vi "Initialize.vi"(8 "error in (no error)":errorcluster, 10 "ConnectParameter":T1, 11 "DataBase in":refnum<class "DataBase.lvclass">) -> (0 "error out":errorcluster, 3 "DataBase out":refnum<class "DataBase.lvclass">)   [LabVIEW 2019, in "DataBase.lvlib" / "DataBase.lvclass"]
uses:
  DataBase.lvclass
  C:/Program Files (x86)/National Instruments/LabVIEW 2019/vi.lib/NI/Event Source Actor/Event Source/Event Source/Event Source.lvclass
  MySQL initial error.lvclass
  C:/Program Files (x86)/National Instruments/LabVIEW 2019/vi.lib/NI/Event Source Actor/Event Source/Event/Event.lvclass
  <vilib>/NI/Event Source Actor/Event Source/Event/Event.lvclass/Event.ctl
  DataBase.lvclass/DataBase.ctl
  <vilib>/addons/database/Connection.llb/DB Tools Open Connec (String).vi
  <vilib>/addons/database/NI_Database_API.lvlib
  <vilib>/NI/Event Source Actor/Event Source/Event/Event.lvclass
  <vilib>/NI/Event Source Actor/Event Source/Event Source/Event Source.lvclass
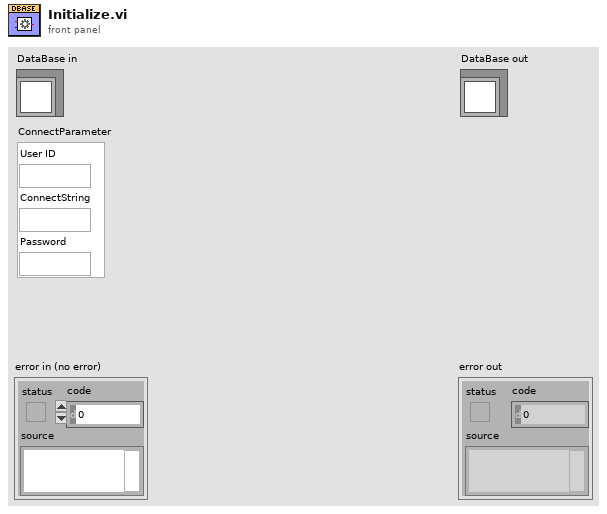
[diagram p1: front panel]
types:
  T1 = cluster{"User ID":string, "ConnectString":string, "Password":string}
  T2 = typedef "NI_Database_API.lvlib/Conn ObjectReference.ctl" = refnum<k1>
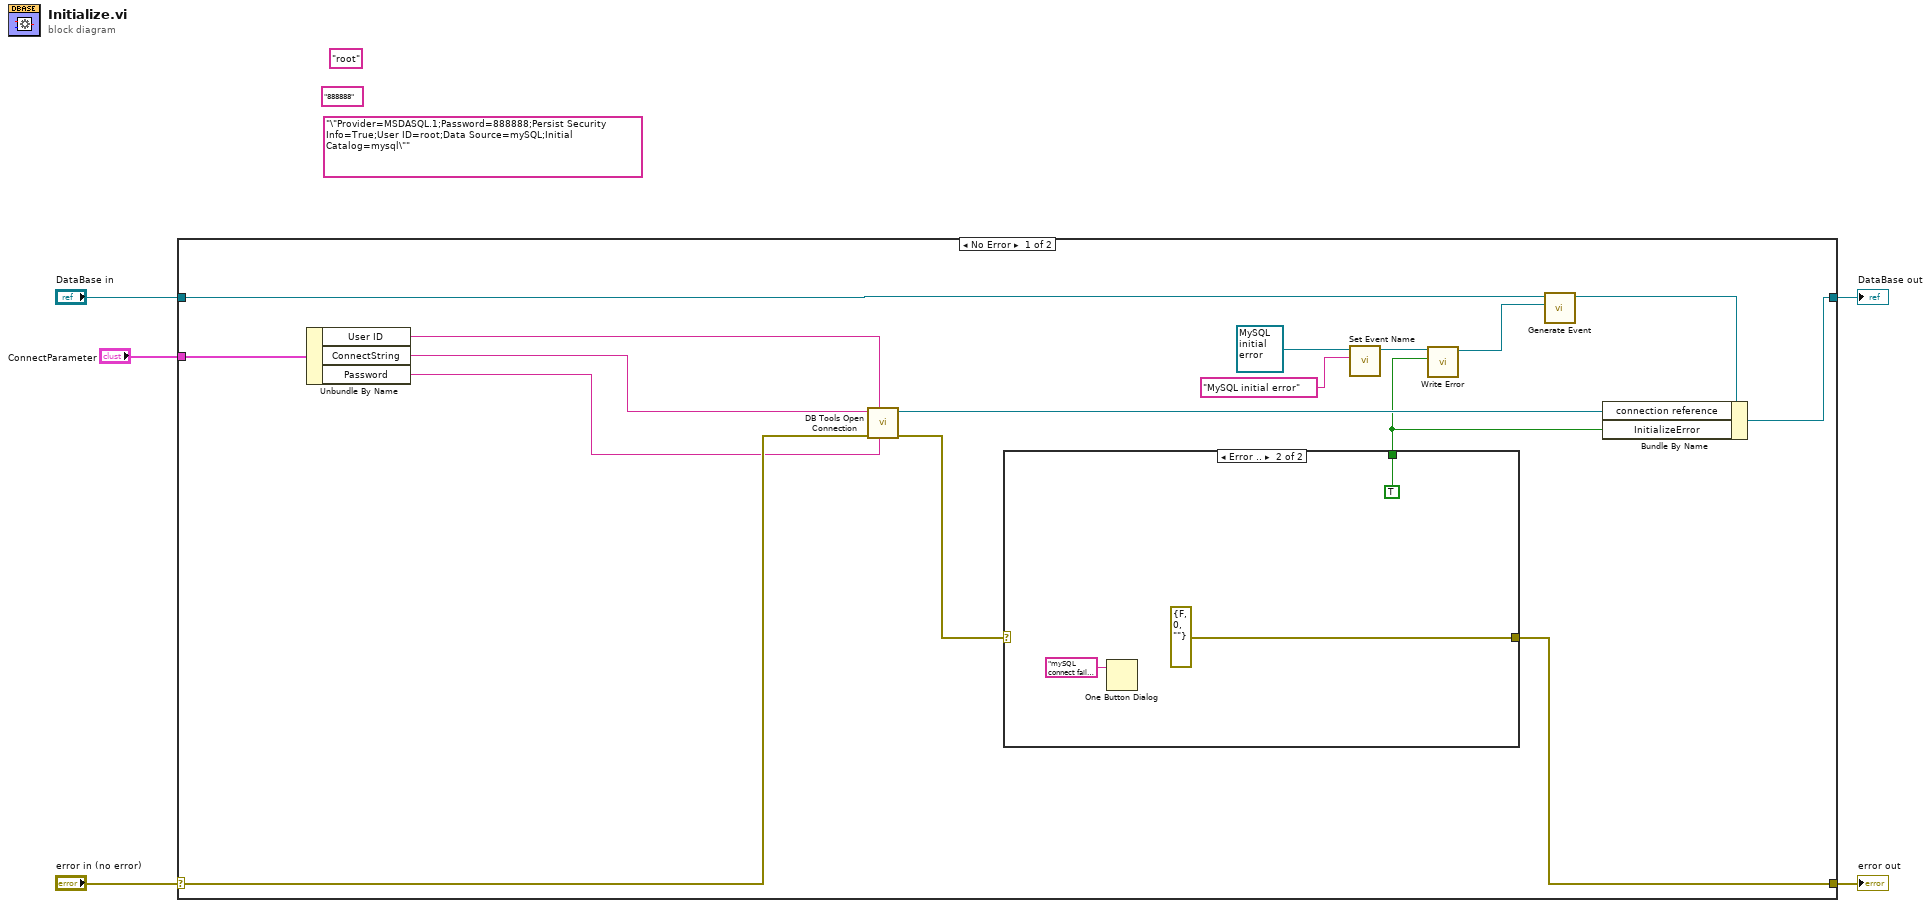
[diagram p0: block diagram]
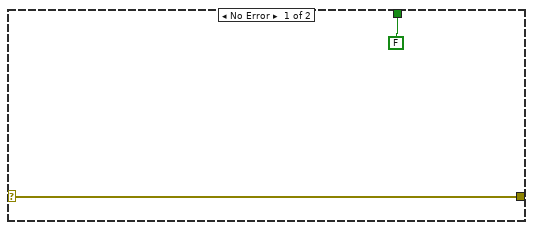
[diagram p2: hidden frame]
diagram:
  (unwired) "root" ("userID")
  (unwired) "888888" ("password")
  (unwired) "\"Provider=MSDASQL.1;Password=888888;Persist Security Info=True;User ID=root;Data Source=mySQL;Initial Catalog=mysql\""
  n1 = case shown="No Error" "error in (no error)" {
    selector: "error in (no error)" -> [w19 w28]
    tunnel: [w13 w28] -> w4
    tunnel: [w20 w27] -> w2
    tunnel: "DataBase in" -> [w8 w27]
    tunnel: "ConnectParameter" -> [w18 _]
    frame No Error {
      n2 = Unbundle By Name(w18) -> ("User ID"=w17:string, "ConnectString"=w16:string, "Password"=w15:string)
      n3 = call-poly <vilib>:"DB Tools Open Connection.vi"("password"=w15, "userID"=w17, "error in (no error)"=w19, "connection information"=w16) -> ("error out"=w14:errorcluster, "connection reference"=w21:T2)  [unwired: 4 in]
      n4 = case shown="Error .." w14 {
        selector: w14 -> [w23 _]
        tunnel: [w23 errorcluster {"status"=FALSE, "code"=0, "source"=""} ("error IO")] -> w13
        tunnel: [FALSE TRUE] -> w6
        frame No Error {
        }
        frame Error {
          n5 = One Button Dialog(message="mySQL connect fail, please check connect parameter!") -> ()  [unwired: 1 in, 1 out]
        }
      }
      n6 = call <vilib>:"Set Event Name.vi"("Name (Generic)"="MySQL initial error", "Event In"=refnum<class "MySQL initial error.lvclass"> refnum ("DataBase.lvlib:MySQL initial erroe.lvclass")) -> ("Event Out"=w11:refnum<class "MySQL initial error.lvclass">)  [unwired: 9 in]
      n7 = call-dynamic "Write Error.vi"("Error"=w6, "MySQL initial erroe in"=w11) -> ("MySQL initial erroe out"=w12:refnum<class "MySQL initial error.lvclass">)  [unwired: 8 in, 1 out]
      n8 = call <vilib>:"Generate Event.vi"("Event"=w12, "Event Source In"=w8) -> ("Event Source Out"=w7:refnum<class "DataBase.lvclass">)  [unwired: 8 in, 1 out]
      n9 = Bundle By Name(cluster=w7, "connection reference"=w21, "InitializeError"=w6) -> (w20:refnum<class "DataBase.lvclass">)
    }
    frame Error {
    }
  }
  "error out" <- w4
  "DataBase out" <- w2
